vi "Flash LED.vi"(0 "MAC Address in Hex":string, 5 "error in (no error)":errorcluster) -> (6 "Flash LED Frame":string, 8 "error out":errorcluster)   [LabVIEW 2017]
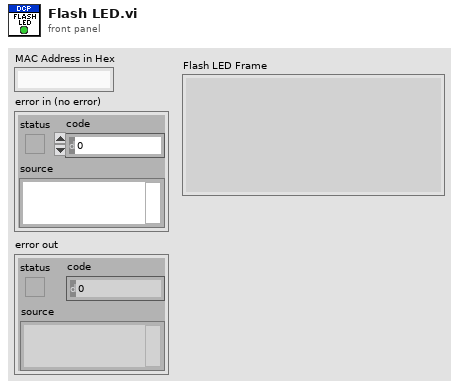
[diagram p1: front panel]
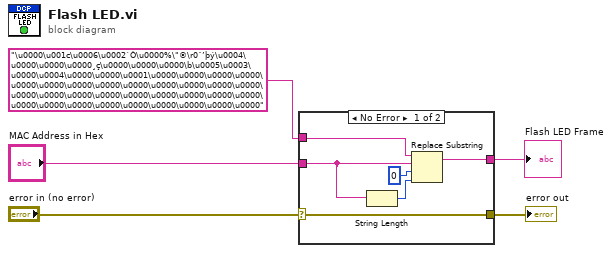
[diagram p0: block diagram]
diagram:
  n1 = case shown="No Error" "error in (no error)" {
    selector: "error in (no error)" -> [w8 w12]
    tunnel: "\u0000\u001c\u0006\u0002`Ò\u0000%\"®\r0ˆ’þý\u0004\u0000\u0000\u0000¸ç\u0000\u0000\u0000\b\u0005\u0003\u0000\u0004\u0000\u0000\u0001\u0000\u0000\u0000\u0000\u0000\u0000\u0000\u0000\u0000\u0000\u0000\u0000\u0000\u0000\u0000\u0000\u0000\u0000\u0000\u0000\u0000\u0000\u0000\u0000\u0000\u0000\u0000\u0000\u0000\u0000\u0000" -> [w10 _]
    tunnel: "MAC Address in Hex" -> [w7 _]
    tunnel: [w9 _] -> w3
    tunnel: [w8 w12] -> w1
    frame No Error {
      n2 = String Length(string=w7) -> (length=w6:i32)
      n3 = Replace Substring(2:w6, 3:0 ("length (len. of substring)"), 4:w7, 5:w10) -> (1:w9:string)  [unwired: 1 out]
    }
    frame Error {
    }
  }
  "Flash LED Frame" <- w3
  "error out" <- w1
